vi "extractTopicName.vi"(8 "error in (no error)":errorcluster, 11 "Module in":refnum<class "Module.lvclass">) -> (0 "error out":errorcluster, 2 "topicName":string, 3 "Module out":refnum<class "Module.lvclass">)   [LabVIEW 2015, in "Module.lvclass"]
uses:
  Module.lvclass
  Module.lvclass/Module.ctl
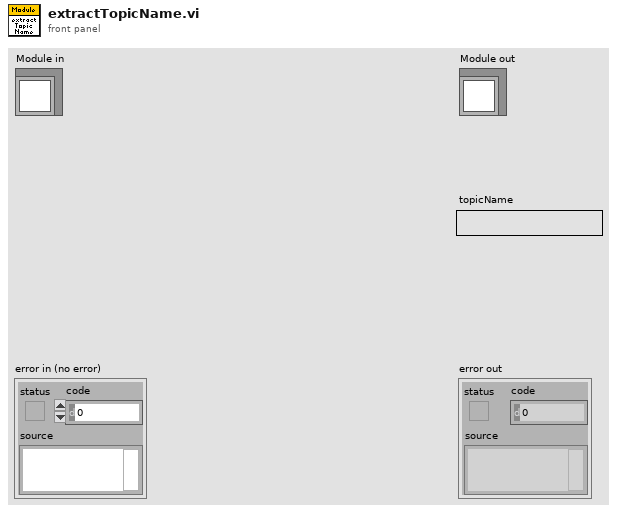
[diagram p1: front panel]
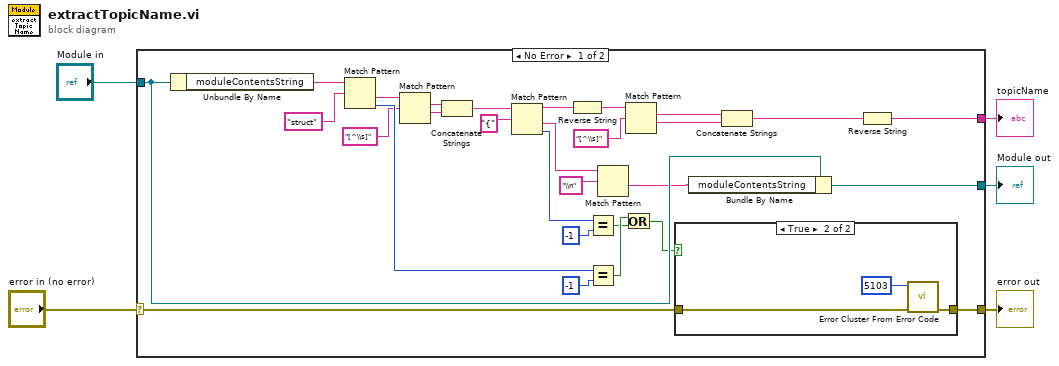
[diagram p0: block diagram]
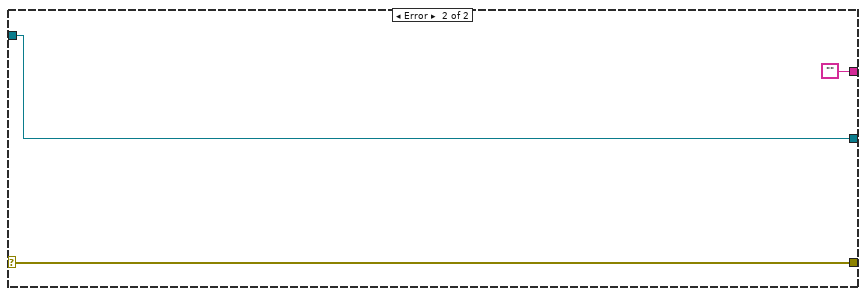
[diagram p3: hidden frame]
diagram:
  n1 = case shown="No Error" "error in (no error)" {
    selector: "error in (no error)" -> [w24 w41]
    tunnel: [w23 w41] -> w4
    tunnel: [w27 w40] -> w2
    tunnel: "Module in" -> [w28 w40]
    tunnel: [w8 ""] -> w1
    frame No Error {
      n2 = Unbundle By Name(w28) -> ("moduleContentsString"=w26:string)
      n3 = Match Pattern(string=w26, regular expression="struct") -> (after substring=w7:string, offset past match=w33:i32)  [unwired: 1 in, 2 out]
      n4 = Match Pattern(string=w7, regular expression="[^\\s]") -> (match substring=w20:string, after substring=w19:string)  [unwired: 1 in, 2 out]
      n5 = Concatenate Strings(w20, w19) -> (w18:string)
      n6 = Match Pattern(string=w18, regular expression="{") -> (before substring=w17:string, after substring=w14:string, offset past match=w6:i32)  [unwired: 1 in, 1 out]
      n7 = Reverse String(1:w17) -> (0:w16:string)
      n8 = Equal?(x=w6, y=-1) -> (x = y?=w29:bool)
      n9 = Equal?(x=w33, y=-1) -> (x = y?=w30:bool)
      n10 = Match Pattern(string=w14, regular expression="\\n") -> (after substring=w9:string)  [unwired: 1 in, 3 out]
      n11 = Or(x=w30, y=w29) -> (x .or. y?=w25:bool)
      n12 = Match Pattern(string=w16, regular expression="[^\\s]") -> (match substring=w12:string, after substring=w11:string)  [unwired: 1 in, 2 out]
      n13 = case shown="True" w25 {
        tunnel: w24 -> [w35 w37]
        tunnel: [w35 w36] -> w23
        frame False {
        }
        frame True {
          n14 = call <vilib>:"Error Cluster From Error Code.vi"("error in (no error)"=w37, "error code (0)"=5103) -> ("error out"=w36:errorcluster)  [unwired: 7 in]
        }
      }
      n15 = Bundle By Name(cluster=w28, "moduleContentsString"=w9) -> (w27:refnum<class "Module.lvclass">)
      n16 = Concatenate Strings(w12, w11) -> (w10:string)
      n17 = Reverse String(1:w10) -> (0:w8:string)
    }
    frame Error {
    }
  }
  "error out" <- w4
  "Module out" <- w2
  "topicName" <- w1
